vi "Tektronix TDS 200 1000 2000 Series Acquire Continuous Waveform.vi"() -> ()   [LabVIEW 2017]
doc: "This example shows how to use autosetup and acquire a waveform on a single channel."
uses:
  <instrlib>/Tektronix TDS 200 1000 2000 Series/Tektronix TDS 200 1000 2000 Series.lvlib
panel:
  in  "Iniciar":bool
  in  "Guardar":bool
  in  "Canal":u16(ring) items=["Channel 1", "Channel 2", "Channel 3", "Channel 4", "Math", "Reference A", "Reference B", "Reference C", "Reference D"]
  in  "stop":bool
  in  "Atenuación de la punta":dbl=1.0
  out "Tektronix TDS 2012B":waveform(dbl)(graph)
  in  "VISA resource name":refnum<visa-resource-name>="Tektronix_TDS2012C"
  # "ENA"
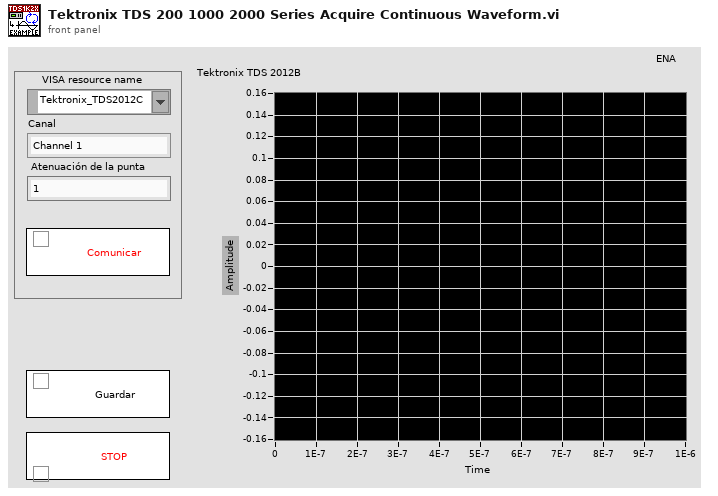
[diagram p1: front panel]
types:
  T1 = enum8{"Enabled", "Disabled", "Disabled and Grayed Out"}
  T2 = cluster{"Baud Rate":u32, "Parity":u16, "Stop Bits":u16, "Flow Control":u16}
  T3 = enum16{"open", "replace", "create", "open or create", "replace or create", "replace or create with confirmation"}
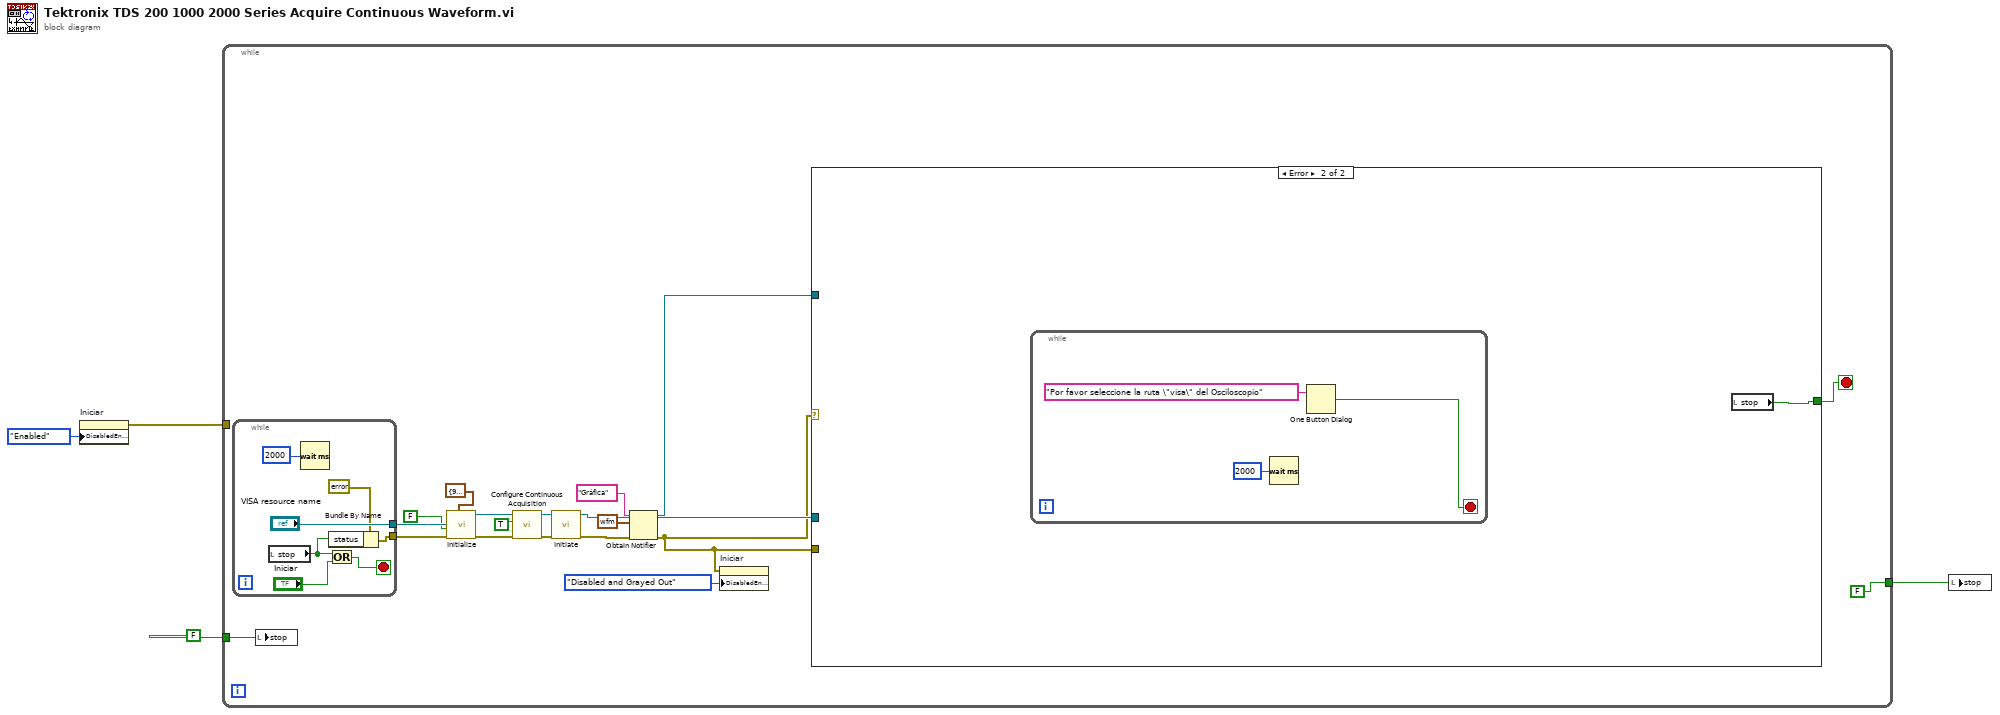
[diagram p0: block diagram]
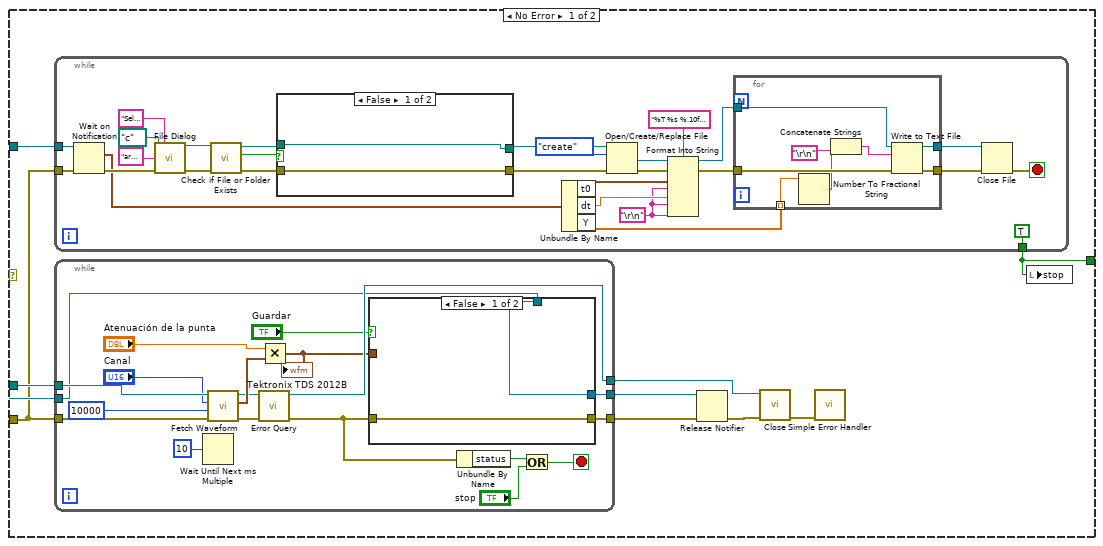
[diagram p2: hidden frame]
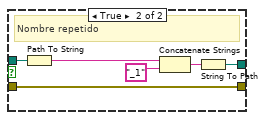
[diagram p3: hidden frame]
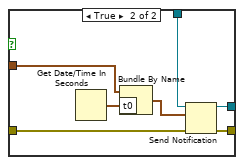
[diagram p4: hidden frame]
diagram:
  n1 = property on="Iniciar" class="Bool"("DisabledEnum"=T1."Enabled" ("Disabled")) -> (error out=w3:errorcluster)  [unwired: 2 in, 1 out]
  n2 = while {
    tunnel: w3 -> [_]
    tunnel: [FALSE ("stop")] -> w2
    tunnel: FALSE ("stop") -> [w6]
    stop <- w5 stop-if-true
    n3 = while {
      tunnel: ["VISA resource name"] -> w23
      tunnel: [w24] -> w7
      stop <- w27 stop-if-true
      n4 = local read "stop"() -> (w26:bool)
      n5 = Wait (ms)(milliseconds to wait=u32 2000) -> ()  [unwired: 1 out]
      n6 = Or(x=w26, y="Iniciar") -> (x .or. y?=w27:bool)
      n7 = Bundle By Name(cluster=errorcluster {"status"=FALSE, "code"=0, "source"=""} ("error in (no error)"), "status"=w26) -> (w24:errorcluster)
    }
    n8 = local write "stop"(w6) -> ()
    n9 = call <instrlib>:"Initialize.vi"("Serial Configuration"=T2 {"Baud Rate"=9600, "Parity"=0, "Stop Bits"=10, "Flow Control"=2}, "error in (no error)"=w7, "Reset? (T: Yes)"=FALSE, "VISA resource name"=w23) -> ("error out"=w15:errorcluster, "VISA resource name out"=w16:refnum<visa-resource-name>)  [unwired: 6 in]
    n10 = call <instrlib>:"Configure Continuous Acquisition.vi"("error in (no error)"=w15, "Enable Continuous Acquisition Mode (True)"=TRUE, "VISA resource name"=w16) -> ("error out"=w20:errorcluster, "VISA resource name out"=w19:refnum<visa-resource-name>)  [unwired: 7 in]
    n11 = call <instrlib>:"Initiate.vi"("error in (no error)"=w20, "VISA resource name"=w19) -> ("error out"=w12:errorcluster, "VISA resource name out"=w18:refnum<visa-resource-name>)  [unwired: 8 in]
    n12 = Obtain Notifier(name (unnamed)="Gráfica", notification data type=waveform(dbl) {"t0"=timestamp(-5.000000000032756e-06 s since 1904-01-01), "dt"=4e-09, "Y"=array[2500 elements]} ("Waveform Data"), error in (no error)=w12) -> (notifier out=w13:refnum<notifier>, error out=w9:errorcluster)  [unwired: 1 in, 1 out]
    n13 = property on="Iniciar" class="Bool"(error in=w9, "DisabledEnum"=T1."Disabled and Grayed Out" ("Disabled")) -> ()  [unwired: 1 in, 2 out]
    n14 = case shown="Error" w9 {
      tunnel: w18 -> [w37 _]
      tunnel: w13 -> [w35 _]
      tunnel: w9 -> [w34 _]
      tunnel: [w31 w112] -> w5
      frame No Error {
        n15 = while {
          tunnel: w35 -> [w67]
          tunnel: w34 -> [w66]
          tunnel: [TRUE] -> w31
          stop <- w42 stop-if-true
          w45 = "\r\n"
          n16 = Wait on Notification(notifier=w67, error in (no error)=w66) -> (notification=w51:waveform(dbl), error out=w65:errorcluster)  [unwired: 2 in, 2 out]
          n17 = call "File Dialog"("start path"=path "c:/", "prompt"="Selecciona por favor el lugar y nombre de tu archivo", "default name"="archivo", "error in"=w65) -> ("selected path"=w61:path, "error out"=w60:errorcluster)  [unwired: 8 in, 2 out]
          n18 = call <vilib>:"Check if File or Folder Exists.vi"("error in (no error)"=w60, "path"=w61) -> ("error out"=w54:errorcluster, "file or folder exists?"=w59:bool, "dup path"=w58:path)  [unwired: 7 in]
          n19 = case shown="False" w59 {
            tunnel: w58 -> [w77 w83]
            tunnel: [w77 w79] -> w57
            tunnel: [w76 w78] -> w55
            tunnel: w54 -> [w76 w78]
            frame False {
            }
            frame True {
              # "Nombre repetido"
              n20 = Path To String(path=w83) -> (string=w82:string)
              n21 = Concatenate Strings(w82, "_1" ("string")) -> (w80:string)
              n22 = String To Path(string=w80) -> (path=w79:path)
            }
          }
          n23 = Unbundle By Name(w51) -> ("t0"=w50:timestamp, "dt"=w49:dbl, "Y"=w47:dbl[])
          n24 = Open/Create/Replace File(file path (use dialog)=w57, error in=w55, operation (0:open)=T3."create") -> (refnum out=w53:refnum<file>, error out=w52:errorcluster)  [unwired: 3 in, 1 out]
          n25 = Format Into String(format string="%T %s %.10f %s %s", initial string=w53, error in=w52, w50, w45, w49, w45, w45) -> (resulting string=w48:refnum<file>, error out=w46:errorcluster)
          n26 = for {
            tunnel: w48 -> [w74]
            tunnel: w47 -> [w73] mode=indexing
            tunnel: w46 -> [w75]
            tunnel: [w69] -> w43
            tunnel: [w68] -> w44
            n27 = Number To Fractional String(number=w73) -> (F-format string=w72:string)  [unwired: 3 in]
            n28 = Concatenate Strings(w72, "\r\n") -> (w71:string)
            n29 = Write to Text File(file (use dialog)=w74, text=w71, error in=w75) -> (refnum out=w68:refnum<file>, error out=w69:errorcluster)  [unwired: 1 in, 1 out]
          }
          n30 = Close File(refnum=w44, error in=w43) -> (error out=w42:errorcluster)  [unwired: 1 out]
        }
        n31 = while {
          tunnel: w37 -> [w102]
          tunnel: w34 -> [w101]
          tunnel: [w93] -> w38
          tunnel: [w84] -> w33
          tunnel: w35 -> [w87]
          tunnel: [w86] -> w36
          stop <- w98 stop-if-true
          n32 = Wait Until Next ms Multiple(millisecond multiple=u32 10) -> ()  [unwired: 1 out]
          n33 = call <instrlib>:"Fetch Waveform.vi"("error in (no error)"=w101, "Timeout (10000 ms)"=u32 10000, "Source (0: Channel 1)"="Canal", "VISA resource name"=w102) -> ("error out"=w95:errorcluster, "Waveform Data"=w100:waveform(dbl), "VISA resource name out"=w94:refnum<visa-resource-name>)  [unwired: 5 in]
          n34 = call <instrlib>:"Error Query.vi"("error in (no error)"=w95, "VISA resource name"=w94) -> ("error out"=w85:errorcluster, "VISA resource name out"=w93:refnum<visa-resource-name>)  [unwired: 6 in, 2 out]
          n35 = Multiply(x="Atenuación de la punta", y=w100) -> (x*y=w88:waveform(dbl))
          "Tektronix TDS 2012B" <- w88
          n36 = case shown="False" "Guardar" {
            tunnel: w88 -> [_ w106]
            tunnel: w87 -> [w104 w111]
            tunnel: [w104 w110] -> w86
            tunnel: w85 -> [w103 w109]
            tunnel: [w103 w108] -> w84
            frame False {
            }
            frame True {
              n37 = Get Date/Time In Seconds() -> (seconds since 1Jan1904=w107:timestamp)
              n38 = Bundle By Name(cluster=w106, "t0"=w107) -> (w105:waveform(dbl))
              n39 = Send Notification(notification=w105, notifier=w111, error in (no error)=w109) -> (notifier out=w110:refnum<notifier>, error out=w108:errorcluster)
            }
          }
          n40 = Unbundle By Name(w85) -> ("status"=w97:bool)
          n41 = Or(x=w97, y="stop") -> (x .or. y?=w98:bool)
        }
        n42 = Release Notifier(notifier=w36, error in (no error)=w33) -> (error out=w32:errorcluster)  [unwired: 1 in, 2 out]
        n43 = call <instrlib>:"Close.vi"("error in (no error)"=w32, "VISA resource name"=w38) -> ("error out"=w39:errorcluster)  [unwired: 9 in]
        n44 = call <vilib>:"Simple Error Handler.vi"("error in (no error)"=w39) -> ()  [unwired: 4 in, 5 out]
        n45 = local write "stop"(w31) -> ()
      }
      frame Error {
        n46 = while {
          stop <- w113 stop-if-true
          n47 = Wait (ms)(milliseconds to wait=u32 2000) -> ()  [unwired: 1 out]
          n48 = One Button Dialog(message="Por favor seleccione la ruta \"visa\" del Osciloscopio") -> (true=w113:bool)  [unwired: 1 in]
        }
        n49 = local read "stop"() -> (w112:bool)
      }
    }
  }
  n50 = local write "stop"(w2) -> ()
